vi "CreateRectangle.vi"(6 "Color":u32(colorbox), 8 "Error In":errorcluster, 9 "b":dbl, 10 "a":dbl) -> (0 "Error Out":errorcluster, 3 "Rectangle Out":refnum<class "Rectangle.lvclass">)   [LabVIEW 2021, in "Rectangle.lvclass"]
doc: "Create a object of rectangle class."
uses:
  Rectangle.lvclass
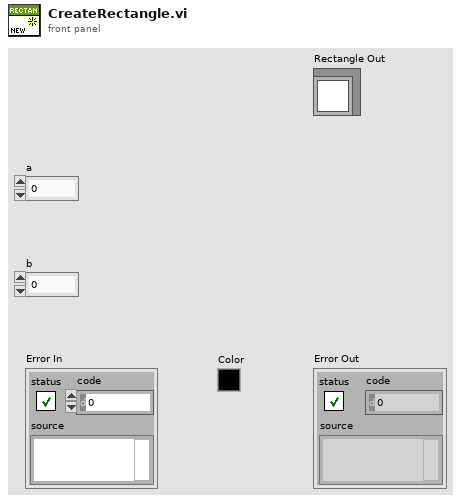
[diagram p1: front panel]
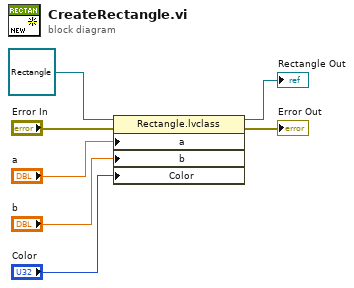
[diagram p0: block diagram]
diagram:
  n1 = property class="Rectangle.lvclass"(reference=refnum<class "Rectangle.lvclass"> refnum ("Rectangle In"), error in="Error In", "a"="a", "b"="b", "Color"="Color") -> (reference out=→"Rectangle Out":refnum<class "Rectangle.lvclass">, error out=→"Error Out":errorcluster)
